vi "erreur.vi"(8 "Données Station Météo":T1, 9 "Thermomètre":dbl(slide) scale=-20.0..50.0) -> (0 "alarme":string, 1 "Alarme temperatutre":bool, 2 "Alarme Pluie":bool, 3 "Alarme Vent":bool, 4 "arret alarme":bool)   [LabVIEW 2017]
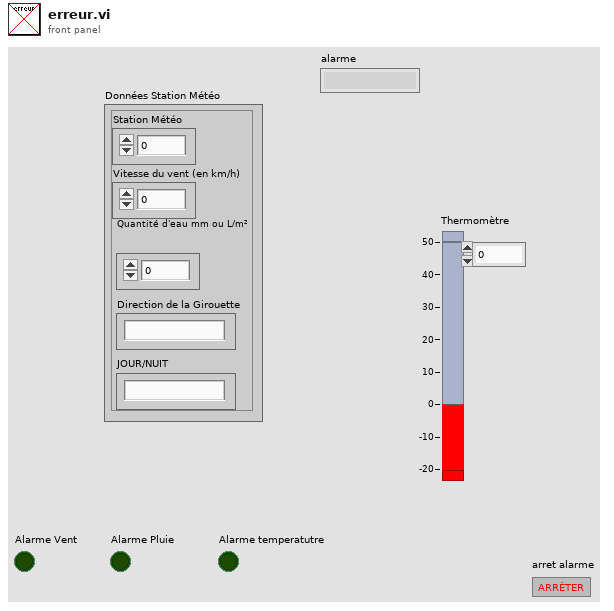
[diagram p1: front panel]
types:
  T1 = cluster{"Station Météo":i32, "Vitesse du vent (en km/h)":dbl, "Quantité d'eau mm ou L/m²":dbl, "Direction de la Girouette":string, "JOUR/NUIT":string}
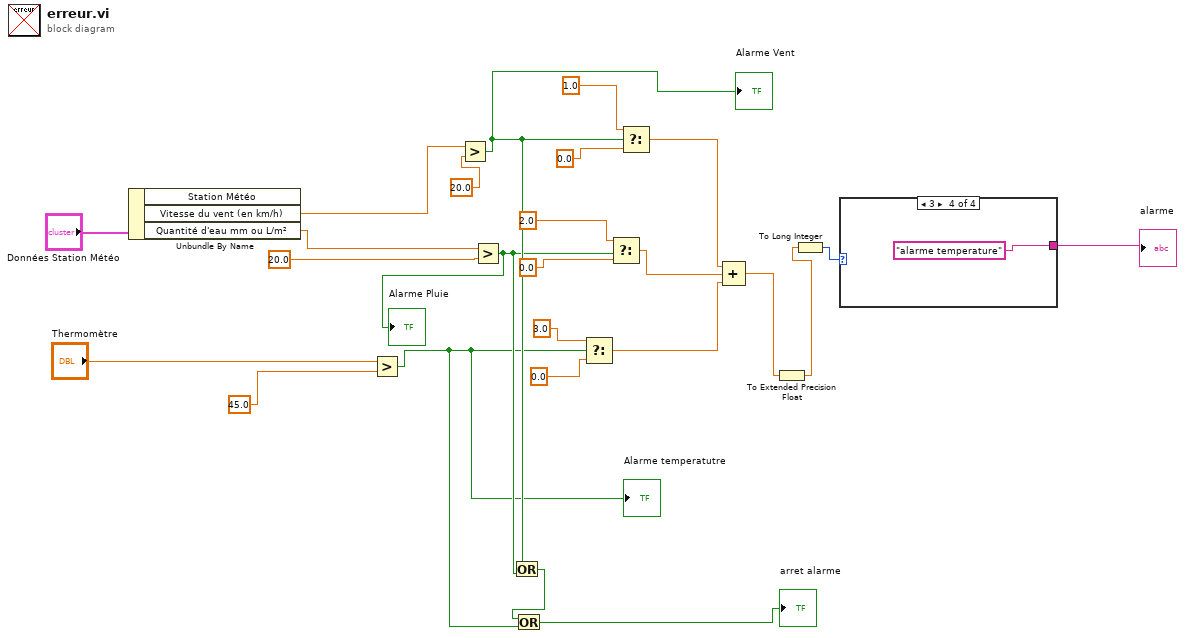
[diagram p0: block diagram]
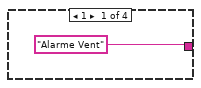
[diagram p2: hidden frame]
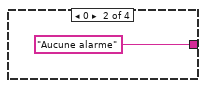
[diagram p3: hidden frame]
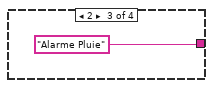
[diagram p4: hidden frame]
diagram:
  n1 = Unbundle By Name("Données Station Météo") -> ("Vitesse du vent (en km/h)"=w23:dbl, "Quantité d'eau mm ou L/m²"=w21:dbl)  [unwired: 1 out]
  n2 = Greater?(x="Thermomètre", y=45.0) -> (0:w2:bool)
  "Alarme temperatutre" <- w2
  n3 = Greater?(x=w23, y=20.0) -> (0:w5:bool)
  "Alarme Vent" <- w5
  n4 = Greater?(x=w21, y=20.0) -> (0:w4:bool)
  "Alarme Pluie" <- w4
  n5 = Or(x=w5, y=w4) -> (x .or. y?=w3:bool)
  n6 = Or(x=w3, y=w2) -> (x .or. y?=→"arret alarme":bool)
  n7 = Select(t=3.0, s=w2, f=0.0) -> (s? t:f=w10:dbl)
  n8 = Select(t=2.0, s=w4, f=0.0) -> (s? t:f=w11:dbl)
  n9 = Select(t=1.0, s=w5, f=0.0) -> (s? t:f=w12:dbl)
  n10 = Compound Arithmetic op=ADD(w12, w11, w10) -> (w9:dbl)
  n11 = To Extended Precision Float(1:w9) -> (0:w7:ext)
  n12 = To Long Integer(number=w7) -> (32bit integer=w8:i32)
  n13 = case shown="3" w8 {
    tunnel: ["Alarme Vent" "Aucune alarme" "Alarme Pluie" "alarme temperature"] -> w6
    frame 1 {
    }
    frame 0 {
    }
    frame 2 {
    }
    frame 3 {
    }
  }
  "alarme" <- w6
